vi "Save Logs.vi"(8 "Error In":errorcluster, 11 "EventLog in":refnum<class "EventLog.lvclass">) -> (0 "Error Out":errorcluster, 3 "EventLog out":refnum<class "EventLog.lvclass">)   [LabVIEW 2019, in "EventLog.lvlib" / "EventLog.lvclass"]
uses:
  EventLog.lvclass
  C:/Projekty/_Wewnetrzne/PC_ActorFramework/07_Program/LABVIEW/02_Source/SubModules/LogsAbstract/LogsAbstract.lvclass
  EventLog.lvclass/EventLog.ctl
  LogsAbstract/LogsAbstract.lvclass/LogsAbstract.ctl
  b2eb4f76-ffae-4243-8d52-1284c2781d6f.vi
  39f41476-d762-4cc0-97d2-8532572a8d36.vi
  39f41476-d762-4cc0-97d2-8532572a8d36.vi/21eb3ad3-1ee9-4327-b564-48b08926d34e.vi
  LogsAbstract/Accessors/Write LogPath.vi
  LogsAbstract/Accessors/Read LogPath.vi
  Classes/Event/Event.lvclass
  C:/Projekty/_Wewnetrzne/PC_ActorFramework/07_Program/LABVIEW/02_Source/Classes/EventsAbstract/EventsAbstract.lvclass
  <vilib>/Utility/Data Type/Get Numeric Information.vi
  <vilib>/Utility/file.llb/Write Delimited Spreadsheet.vi
  <vilib>/Utility/file.llb/Write Delimited Spreadsheet (string).vi
  Classes/EventsAbstract/EventsAbstract.lvclass
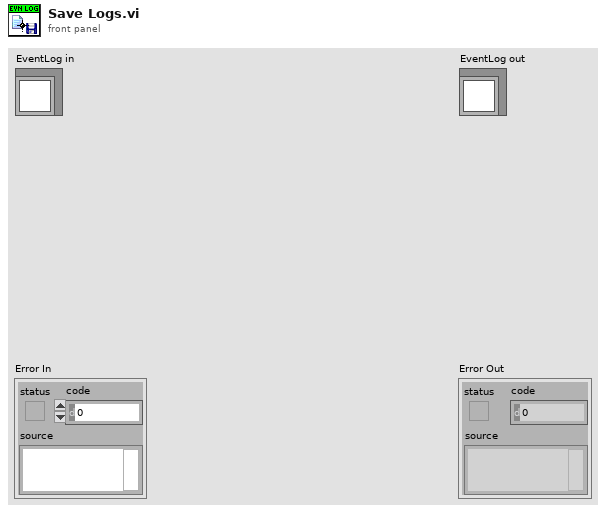
[diagram p1: front panel]
types:
  T1 = typedef "Event.lvclass/Event Classification.ctl" = enum16{"System Log", "test1", "test2", "test3"}
  T2 = cluster{"Date":string, "Time":string, "Description":string, "Comments":string, "Source":string}
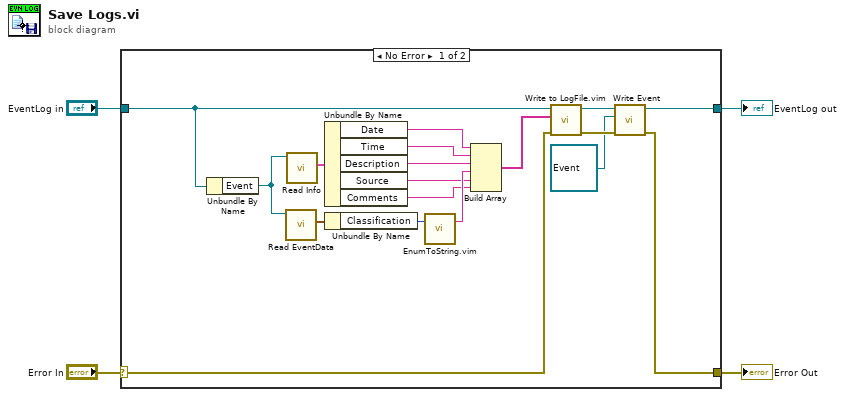
[diagram p0: block diagram]
diagram:
  n1 = case shown="No Error" "Error In" {
    selector: "Error In" -> [w21 w24]
    tunnel: [w8 w24] -> w4
    tunnel: [w6 w23] -> w3
    tunnel: "EventLog in" -> [w22 w23]
    frame No Error {
      n2 = Unbundle By Name(w22) -> ("Event"=w18:refnum<class "Event.lvclass">)
      n3 = call "Read EventData.vi"("Event in"=w18) -> ("EventData"=w16:cluster{"Classification":T1})  [unwired: 8 in, 2 out]
      n4 = call "Read Info.vi"("EventsAbstract in"=w18) -> ("Info"=w17:T2)  [unwired: 8 in, 2 out]
      n5 = Unbundle By Name(w17) -> ("Date"=w14:string, "Time"=w13:string, "Description"=w12:string, "Source"=w9:string, "Comments"=w10:string)
      n6 = Unbundle By Name(w16) -> ("Classification"=w15:T1)
      n7 = call "EnumToString.vim"("Enum"=w15) -> ("Enum Value"=w11:string)  [unwired: 16 in, 2 out]
      n8 = Build Array(w14, w13, w12, w11, w9, w10) -> (w19:string[])
      n9 = call "Write to LogFile.vim"("Error In"=w21, "Data"=w19, "LogClass In"=w22) -> ("Error out"=w20:errorcluster, "LogClass Out"=w7:refnum<class "EventLog.lvclass">)  [unwired: 7 in]
      n10 = call "Write Event.vi"("error in (no error)"=w20, "Event.lvclass"=refnum<class "Event.lvclass"> refnum, "EventLog in"=w7) -> ("error out"=w8:errorcluster, "EventLog out"=w6:refnum<class "EventLog.lvclass">)  [unwired: 7 in]
    }
    frame Error {
    }
  }
  "Error Out" <- w4
  "EventLog out" <- w3
